vi "Klinger SetZero.vi"(0 "Address GPIB":string="6", 1 "Position Ref":refnum<vi>, 2 "Axe":u8(ring) items=["W", "X", "Y", "Z"], 3 "error in":errorcluster, 4 "UnitDem":u8(ring)=2 caption="Unités" items=["Pas", "mm", "ps"]) -> (5 "Statut":bool, 6 "Ind Comm":string, 7 "error out":errorcluster)   [LabVIEW 2010]
doc: "Ce Vi définit la position actuelle de l'axe spécifié comme zéro."
panel:
  out "Message D'erreur":string
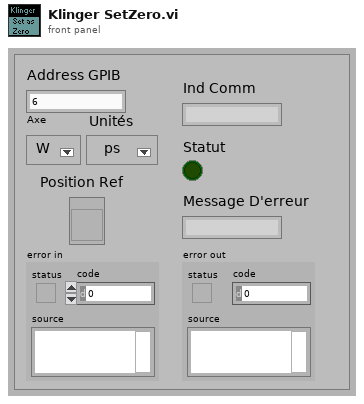
[diagram p1: front panel]
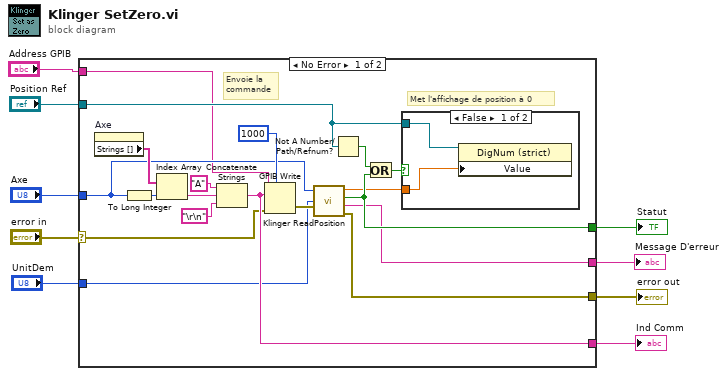
[diagram p0: block diagram]
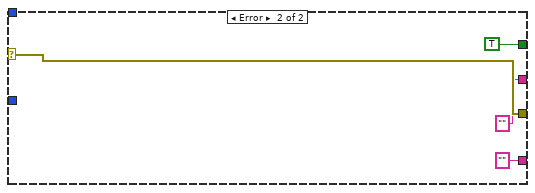
[diagram p3: hidden frame]
diagram:
  n1 = case shown="No Error" "error in" {
    selector: "error in" -> [w16 w34]
    tunnel: [w28 ""] -> w9
    tunnel: "Axe" -> [w13 _]
    tunnel: "Position Ref" -> [w20 _]
    tunnel: [w17 TRUE ("Statut")] -> w6
    tunnel: [w14 w34] -> w5
    tunnel: [w15 "" ("Message D'erreur")] -> w4
    tunnel: "Address GPIB" -> [w11 _]
    tunnel: "UnitDem" -> [w10 _]
    frame No Error {
      # "Envoie la \ncommande"
      # "Met l'affichage de position à 0"
      n2 = property on="Axe" class="Ring (strict)"() -> ("Strings []"=w25:string[])  [unwired: 2 in, 2 out]
      n3 = To Long Integer(number=w13) -> (32bit integer=w24:i32)
      n4 = Index Array(array=w25, index=w24) -> (element=w23:string)
      n5 = Concatenate Strings("A", w23, "\r\n") -> (w28:string)
      n6 = GPIB Write(0:w11, 1:w28, 3:w16, 4:1000 ("timeout ms (488.2 global)")) -> (6:w18:errorcluster)  [unwired: 1 in, 1 out]
      n7 = call <userlib>:"Klinger ReadPosition.vi"("Axe"=w13, "UnitDem"=w10, "error in"=w18) -> ("Position"=w12:dbl, "Statut"=w17:bool, "Cont Error"=w15:string, "error out"=w14:errorcluster)  [unwired: 1 in, 3 out]
      n8 = Not A Number/Path/Refnum?(number/path/refnum=w20) -> (NaN/Path/Refnum?=w19:bool)
      n9 = Or(x=w19, y=w17) -> (x .or. y?=w21:bool)
      n10 = case shown="False" w21 {
        tunnel: w20 -> [w30 _]
        tunnel: w12 -> [w29 _]
        frame False {
          n11 = property class="DigNum (strict)"(reference=w30, "Value"=w29) -> ()  [unwired: 1 in, 2 out]
        }
        frame True {
        }
      }
    }
    frame Error {
    }
  }
  "error out" <- w5
  "Ind Comm" <- w9
  "Message D'erreur" <- w4
  "Statut" <- w6
